vi "运维调试_氨氮.vi"() -> ()   [LabVIEW 2016, in "斯坦道氨氮.lvlib"]
uses:
  <vilib>/Utility/miscctls.llb/LVPointTypeDef.ctl
  <vilib>/Utility/config.llb/NI_LVConfig.lvlib
  <vilib>/ptbypt/NI_PtbyPt.lvlib
panel:
  in  "模块启用":bool
  in  "串口设置":bool
  in  "备用系数一键写入":bool
  in  "公式一键写入":bool
  in  "流程文件路径":path=path "C:/Users/Hsiao/Documents/斯坦道流程文件/流程.xml"
  in  "曲线模型":cluster{"X^2":dbl, "X":dbl, "B":dbl}(xcontrol)
  in  "质控参数设置":bool
  out "字符串":string
  in  "氨氮自动测试量程配置":T1
  out "ADC":sgl
  out "温度2":sgl
  out "温度1":sgl
  out "固件版本号":string
  in  "数组":string[](array[string])
  in  "备用系数写入":bool
  in  "备用系数读取":bool
  in  "备用系数":T2
  in  "量程切换阈值写入":bool
  in  "量程切换阈值读取":bool
  in  "量程切换阈值":cluster{"阈值":dbl, "标液浓度":dbl}
  in  "参数下拉列表":enum16{"氨氮", "总磷"}(ring)
  in  "量程下拉列表":enum16{"低量程", "高量程"}(ring)
  in  "测量模式下拉列表":enum16{"水样测量", "空白核查", "跨度核查", "标样核查", "加标回收"}(ring)
  in  "公式":cluster{"X^2":dbl, "X":dbl, "b":dbl}
  in  "写公式":bool
  in  "读公式":bool
  in  "返回":bool
  in  "设置":bool
  out "序列号":string="序列号"
  out "氨氮测量数据":T3(xcontrol)
  out "集成报警信息":string
  out "定时启动":bool
  out "总磷总氮运行状态":T4(xcontrol)
  in  "停止":bool
  in  "手动启动":bool
  in  "单步测试":bool
  in  "总磷氨氮调试":u16[](xcontrol)
  out "F3":sgl format="%#.6f"
  out "F2":sgl format="%#.6f"
  out "F1":sgl format="%#.6f"
  out "F0":sgl format="%#.6f"
  out "多列列表框":i32(listbox)
  # "参数设置"
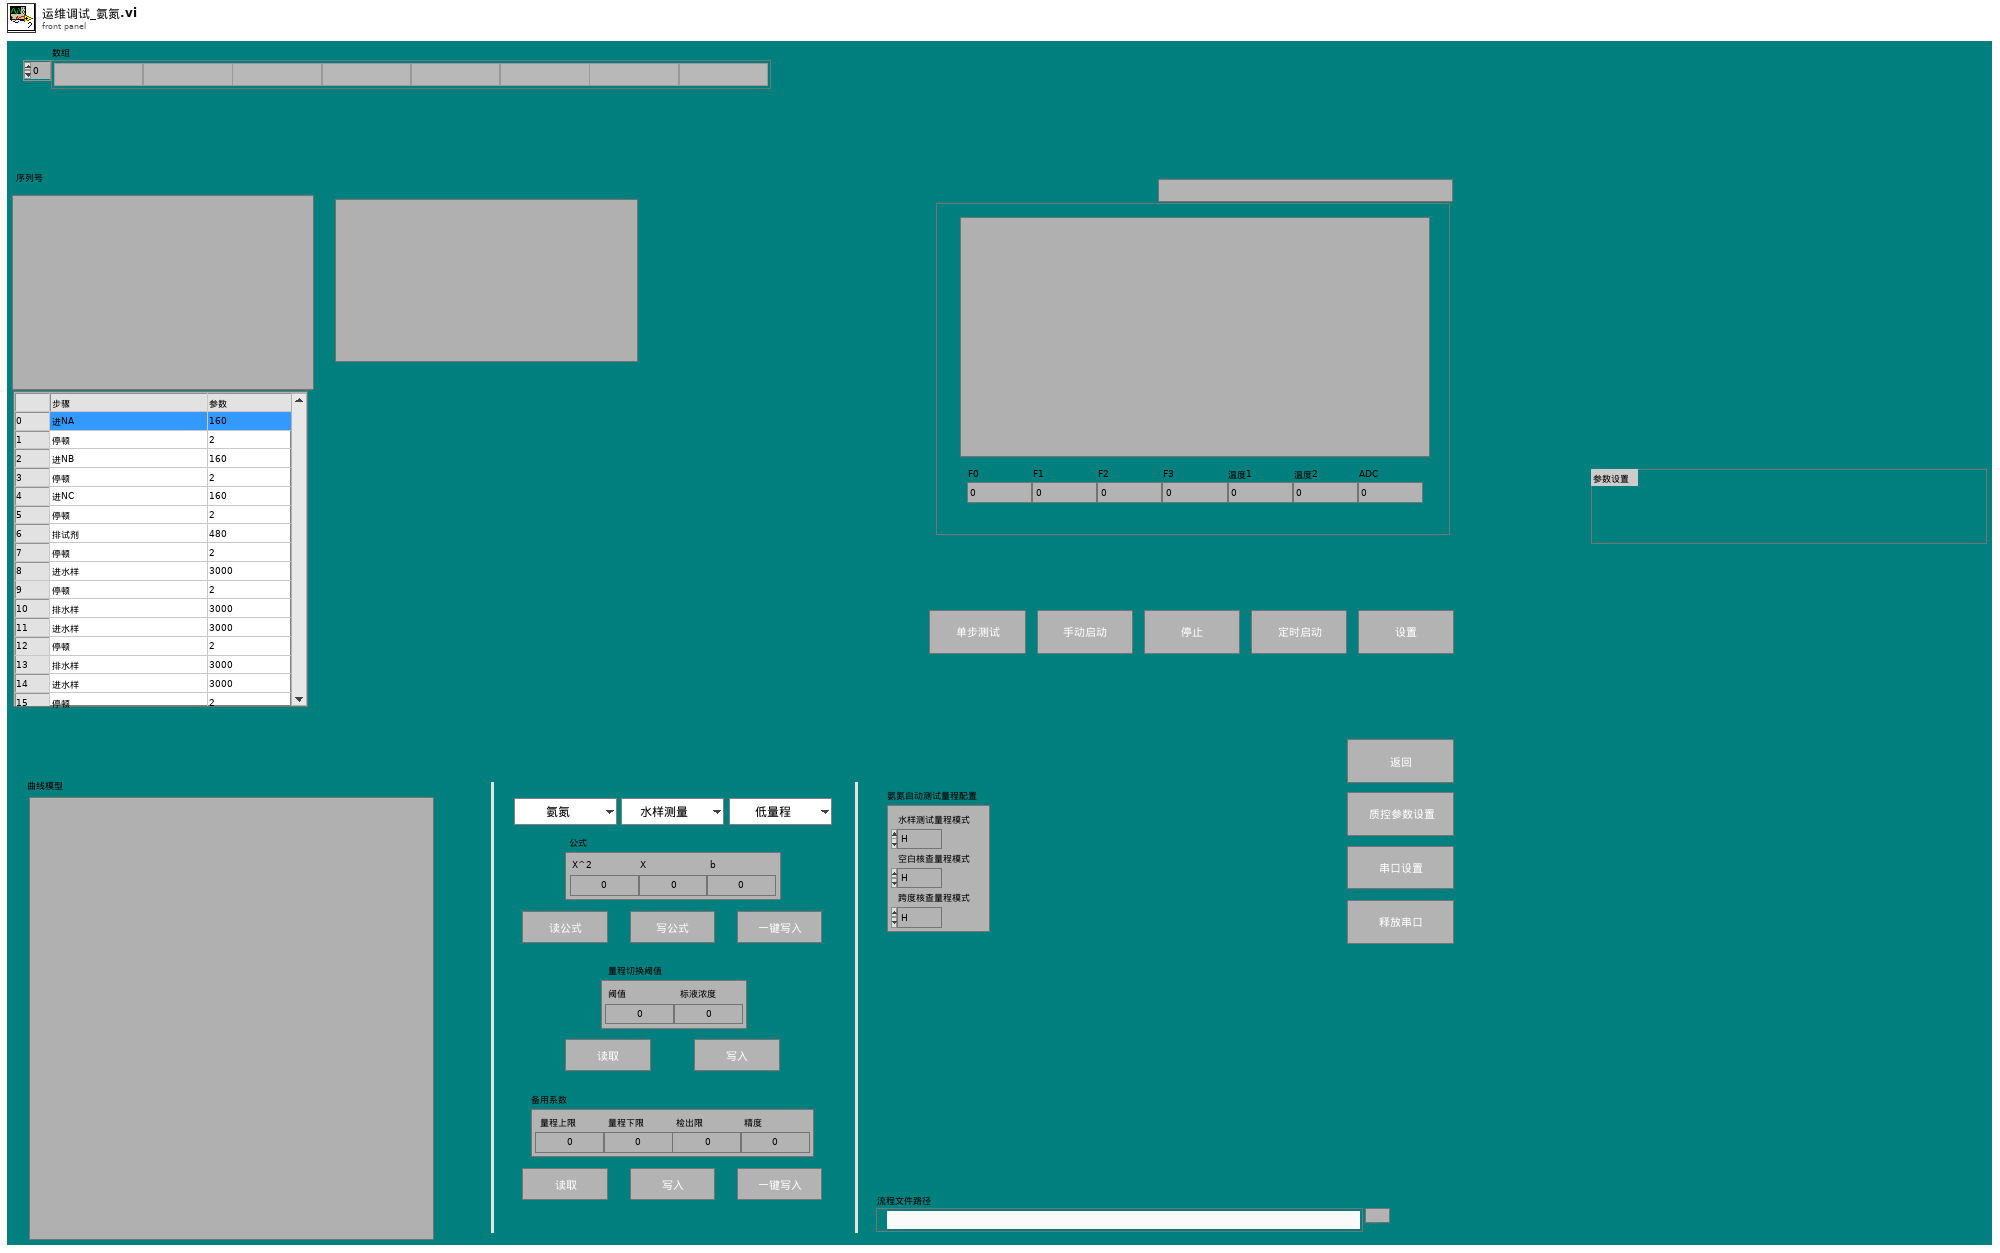
[diagram p1: front panel]
types:
  T1 = cluster{"水样测试量程模式":enum16{"H", "L", "AUTO"}, "空白核查量程模式":enum16{"H", "L", "AUTO"}, "跨度核查量程模式":enum16{"H", "L", "AUTO"}}
  T2 = cluster{"量程上限":dbl, "量程下限":dbl, "检出限":dbl, "精度":dbl}
  T3 = cluster{"flowid":u16, "测量精度":u16, "测量数据区":cluster{"因子编码":u32, "单位":u16, "标样参考值":sgl, "水样数据时间":timestamp, "水样实测值":sgl, "水样数据标识":string, "标样数据时间":timestamp, "标样实测值":sgl, "标样数据标识":string, "空白数据时间":timestamp, "空白实测值":sgl, "空白数据标识":string, "零点核查数据时间":timestamp, "零点核查实测值":sgl, "零点核查数据标识":string, "跨度核查数据时间":timestamp, "跨度核查实测值":sgl, "跨度核查数据标识":string, "加标回收数据时间":timestamp, "加标回收实测值":sgl, "加标回收数据标识":string, "平行样数据时间":timestamp, "平行样实测值":sgl, "平行样数据标识":string}}
  T4 = cluster{"系统时间":timestamp, "工作状态":enum16{"空闲", "水样测试", "标样核查", "零点核查", "跨度核查", "空白测试", "平行样测试", "加标回收", "空白校准", "标样校准", "初始化（清洗）"}, "测量模式":enum16{"待机", "连续模式", "周期模式", "定点模式", "受控模式", "手动模式"}, "告警代码":enum16{"无告警", "缺试剂告警", "缺水样告警", "缺蒸馏水告警", "缺标液告警", "仪表漏液告警", "标定异常告警", "超量程告警", "加热异常", "低试剂预警", "超上限告警", "超下限告警", "仪表内部其他异常", "滴定异常告警", "电极异常告警", "量程切换告警", "参数设置告警", "PH电极电位异常", "电导率电极异常", "浊度光度异常", "溶解氧电极异常", "溶解氧光强异常", "温度异常告警", "PH异常告警", "溶解氧异常告警", "电导率异常告警", "浊度异常告警", "叶绿素异常告警", "藻密度异常告警", "蓝绿藻异常告警", "ORP异常告警", "氨氮异常告警", "清洁刷异常告警", "SD卡异常告警", "蓝牙异常告警", "Wifi异常告警", "流程异常告警"}, "故障代码":enum16{"无故障", "电机故障", "温度故障", "通讯故障", "滴定故障"}, "日志代码":u16, "软件版本":u16, "F0":sgl, "F1":sgl, "F2":sgl, "F3":sgl, "T":sgl, "H":sgl, "id":u16, "flowid":u16, "量程":u16, "总磷控温温度1":sgl, "营养盐控温温度2":sgl, "ADC":sgl}
  T5 = cluster{"站号":u16, "量程切换":enum32{"H", "L", "AUTO"}, "控制命令":enum16{"启动测量", "标样核查", "零点核查", "跨度核查", "空白测试", "平行样测试", "加标回收", "空白校准", "标样校准", "初始化（清洗）", "停止测试", "仪器重启", "校时", "模式设置", "测量间隔设置"}, "模式设置":enum16{"待机", "连续模式", "周期模式", "定点模式", "受控模式", "手动模式"}, "测量间隔":u16}
  T6 = enum16{"启动测量", "标样核查", "零点核查", "跨度核查", "空白测试", "平行样测试", "加标回收", "空白校准", "标样校准", "初始化（清洗）", "停止测试", "仪器重启", "校时", "模式设置", "测量间隔设置"}
  T7 = cluster{"仪器测试类型":enum16{"水样测试", "标样核查", "空白测试", "跨度核查"}, "周期设置类型":enum16{"定点启动", "间隔启动"}, "定时功能启用":bool, "定时间隔":dbl, "24H周期设置":bool[]}
  T8 = enum32{"Bad", "Idle", "Run top level", "Running"}
  T9 = typedef "LVDateTimeRec.ctl" = cluster{"秒数的小数部分":dbl, "秒":i32, "分":i32, "时":i32, "日":i32, "月":i32, "年":i32, "天数（周）":i32, "天数（年）":i32, "DST":i32}
  T10 = typedef "LVPointTypeDef.ctl" = cluster{"Horizontal":i16, "Vertical":i16}
  T11 = cluster{"因子编码":u32, "单位":u16, "标样参考值":sgl, "水样数据时间":timestamp, "水样实测值":sgl, "水样数据标识":string, "标样数据时间":timestamp, "标样实测值":sgl, "标样数据标识":string, "空白数据时间":timestamp, "空白实测值":sgl, "空白数据标识":string, "零点核查数据时间":timestamp, "零点核查实测值":sgl, "零点核查数据标识":string, "跨度核查数据时间":timestamp, "跨度核查实测值":sgl, "跨度核查数据标识":string, "加标回收数据时间":timestamp, "加标回收实测值":sgl, "加标回收数据标识":string, "平行样数据时间":timestamp, "平行样实测值":sgl, "平行样数据标识":string}
  T12 = enum16{"空闲", "水样测试", "标样核查", "零点核查", "跨度核查", "空白测试", "平行样测试", "加标回收", "空白校准", "标样校准", "初始化（清洗）"}
  T13 = typedef "NI_LVConfig.lvlib/Config Data RefNum.ctl" = refnum<k1>
  T14 = cluster{"启动模式":enum16{"跨度核查", "水样测量", "空白核查", "标样核查", "加标回收"}, "启动参数":u16, "量程":enum16{"低量程", "高量程"}}
  T15 = cluster{"时间标识":timestamp, "设备":string, "日志信息":string, "流程参数":string}
  T16 = cluster{"时间标识":timestamp, "设备":string, "日志信息":string}
  T17 = enum16{"无告警", "缺试剂告警", "缺水样告警", "缺蒸馏水告警", "缺标液告警", "仪表漏液告警", "标定异常告警", "超量程告警", "加热异常", "低试剂预警", "超上限告警", "超下限告警", "仪表内部其他异常", "滴定异常告警", "电极异常告警", "量程切换告警", "参数设置告警", "PH电极电位异常", "电导率电极异常", "浊度光度异常", "溶解氧电极异常", "溶解氧光强异常", "温度异常告警", "PH异常告警", "溶解氧异常告警", "电导率异常告警", "浊度异常告警", "叶绿素异常告警", "藻密度异常告警", "蓝绿藻异常告警", "ORP异常告警", "氨氮异常告警", "清洁刷异常告警", "SD卡异常告警", "蓝牙异常告警", "Wifi异常告警", "流程异常告警"}
  T18 = typedef "LVRowAndColumnUnsignedTypeDef.ctl" = cluster{"Row":u32, "Column":u32}
  T19 = cluster{"跨度值":dbl, "零点标准液浓度":dbl, "跨度标准液浓度":dbl, "标准液标准浓度":dbl}
  T20 = cluster{"确定":bool, "跨度值":dbl, "零点标准液浓度":dbl, "跨度标准液浓度":dbl, "标准液标准浓度":dbl}
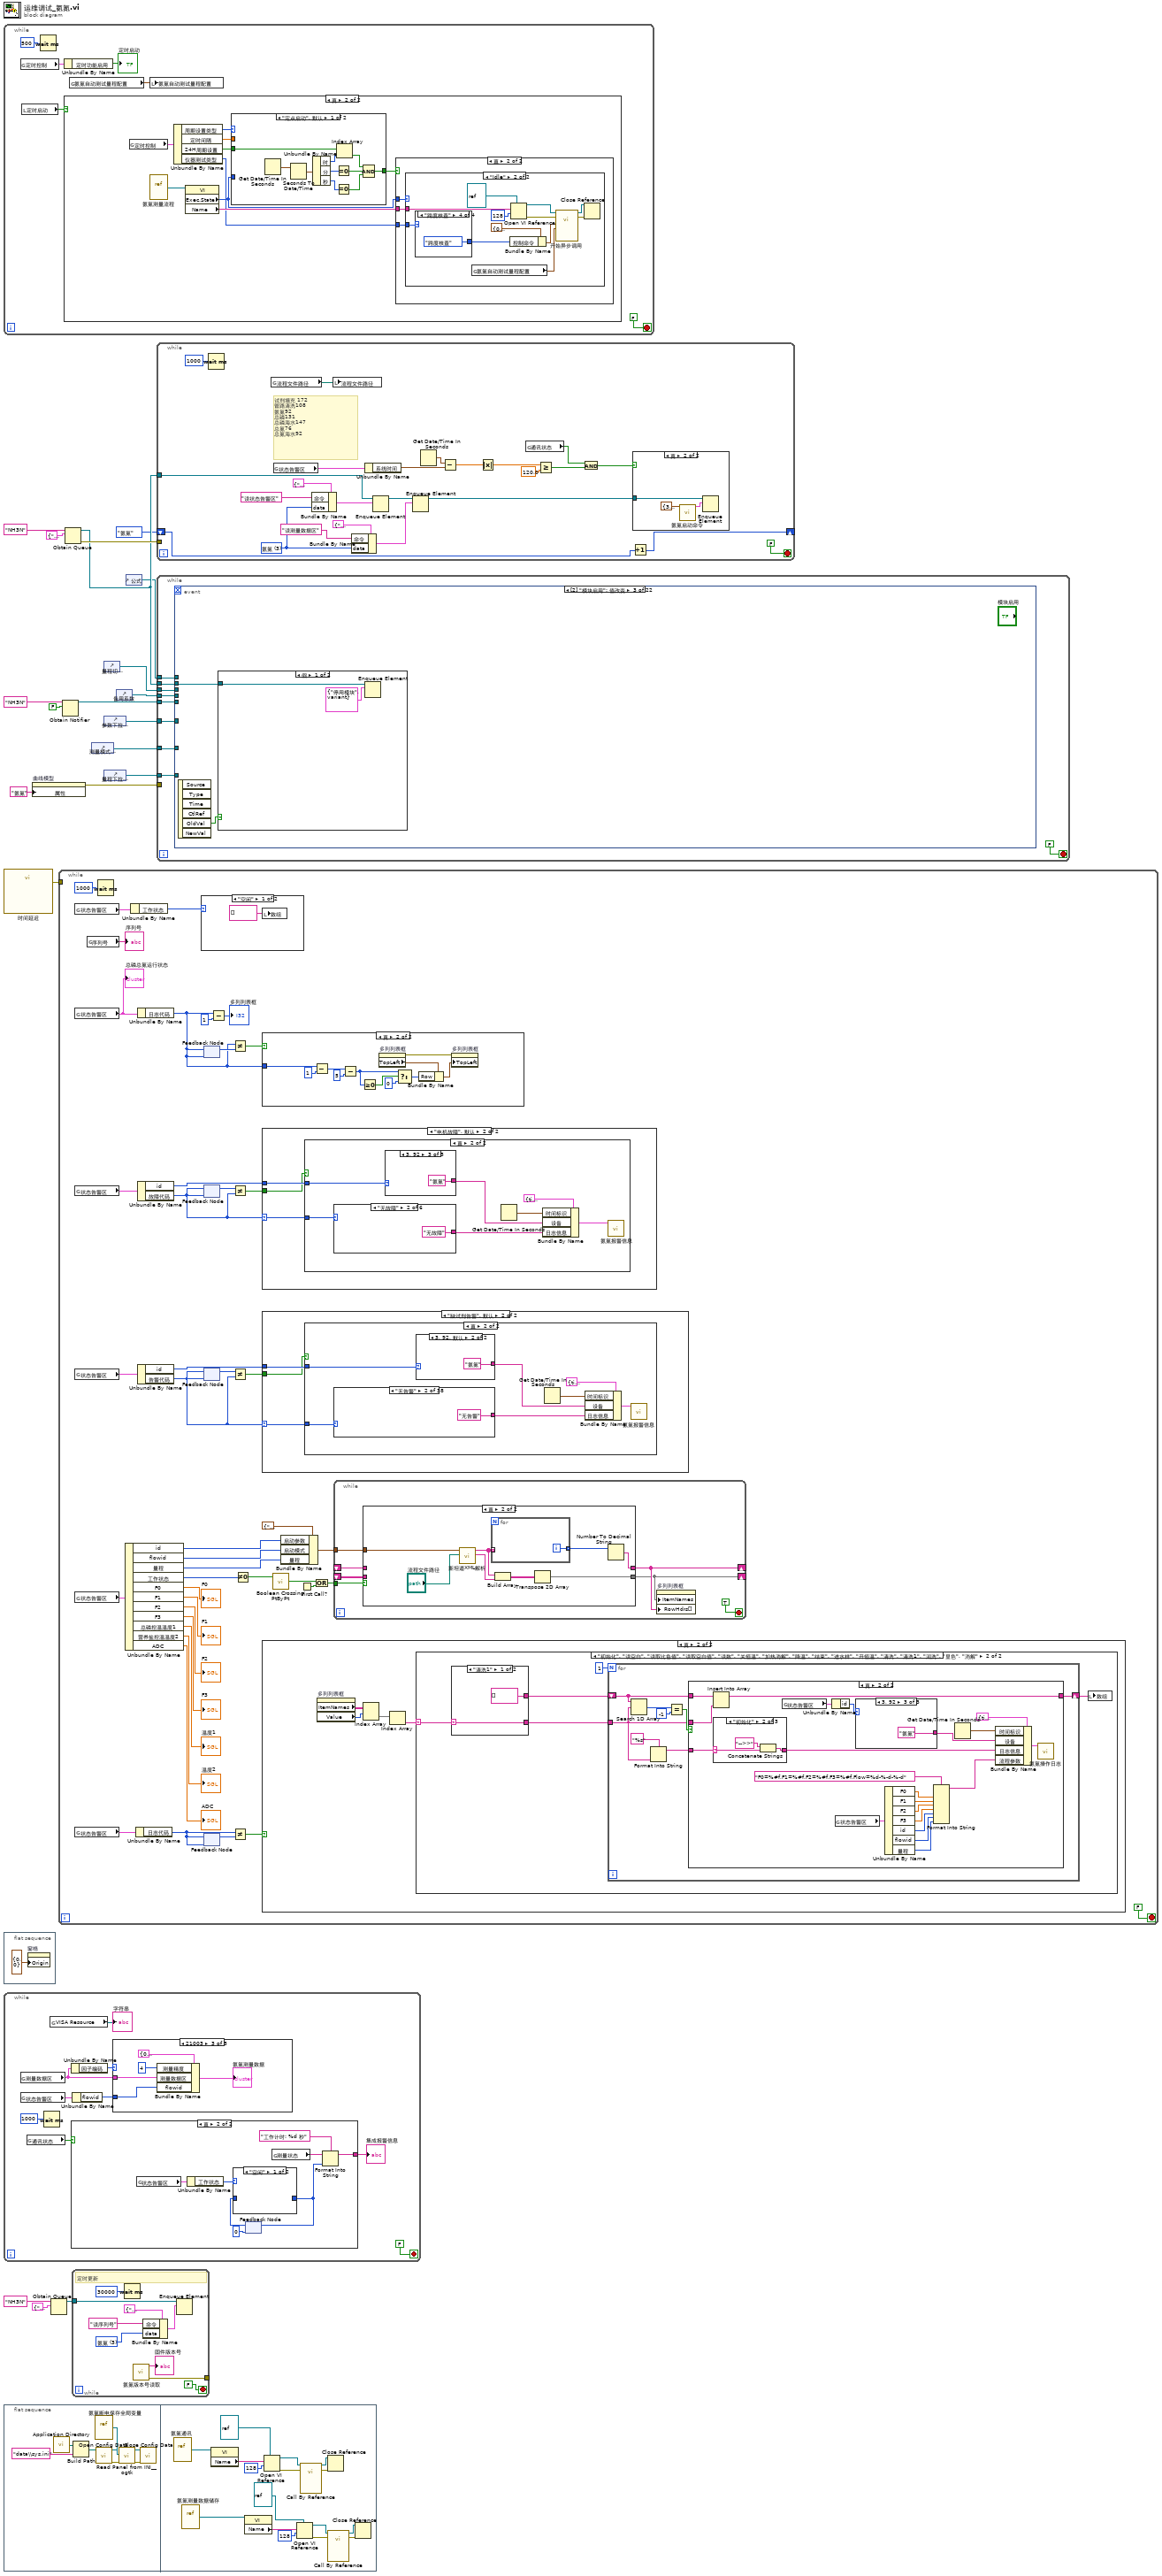
[diagram p0: block diagram]
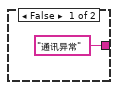
[diagram p2: hidden frame]
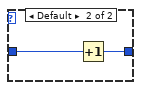
[diagram p3: hidden frame]
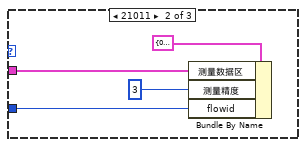
[diagram p5: hidden frame]
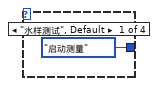
[diagram p9: hidden frame]
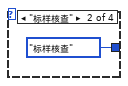
[diagram p10: hidden frame]
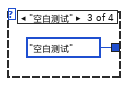
[diagram p11: hidden frame]
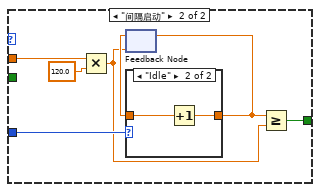
[diagram p12: hidden frame]
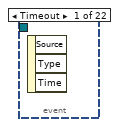
[diagram p14: hidden frame]
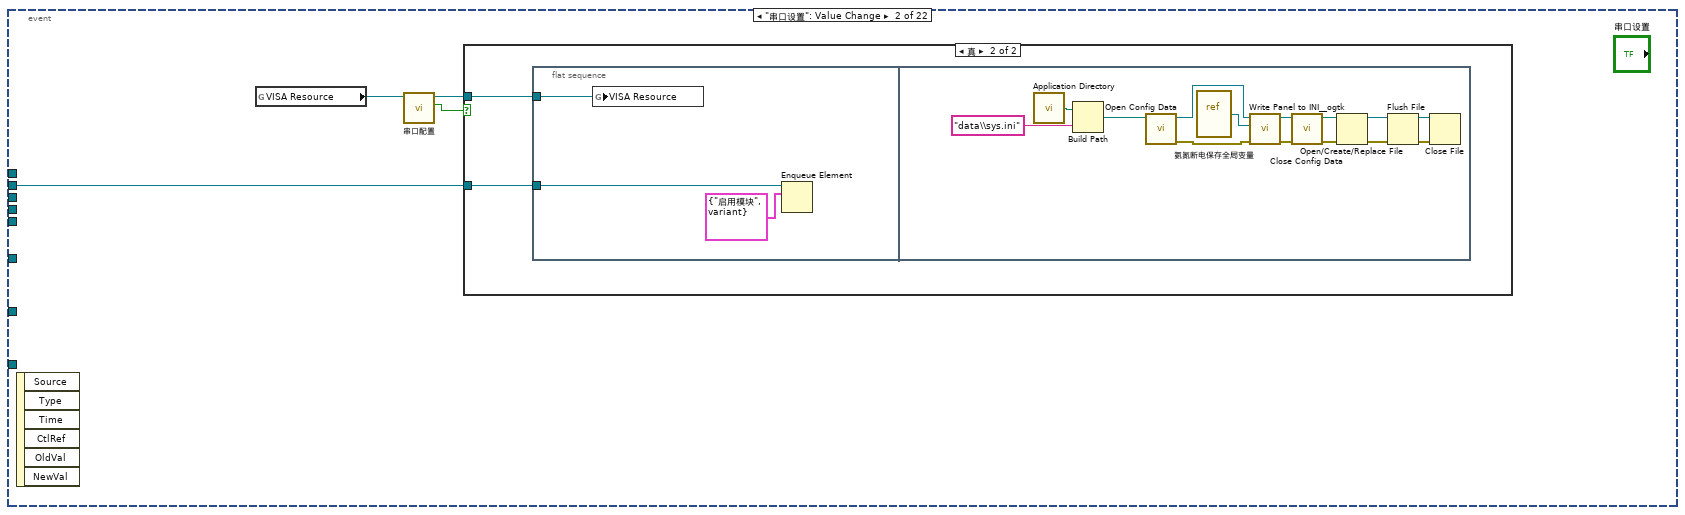
[diagram p15: hidden frame]
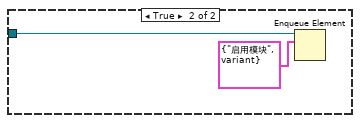
[diagram p17: hidden frame]
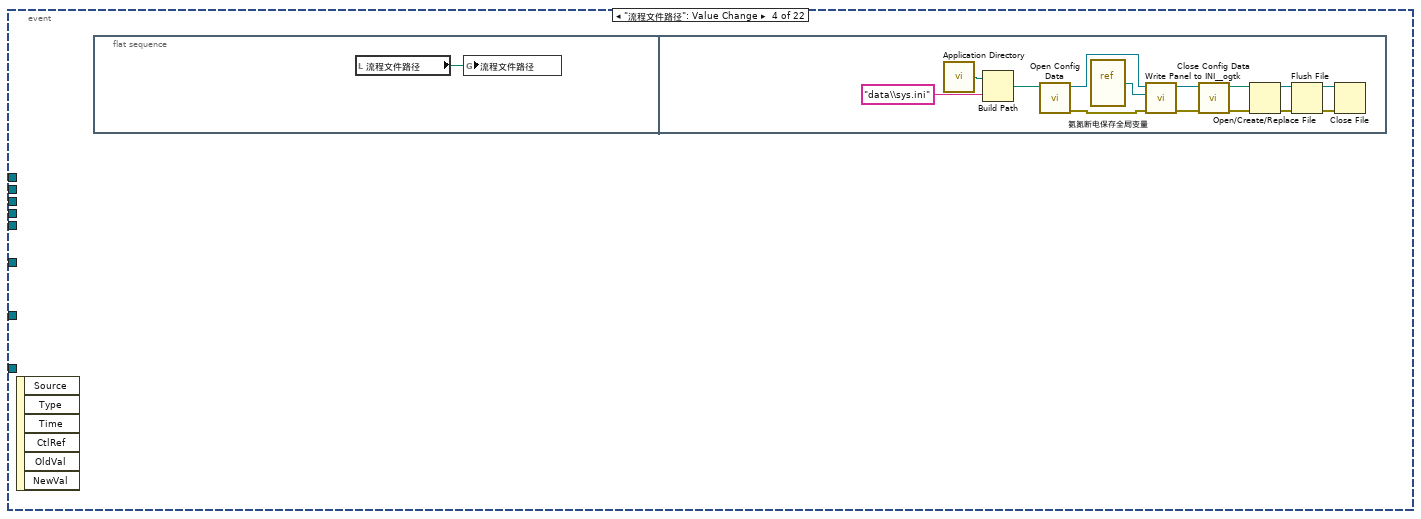
[diagram p18: hidden frame]
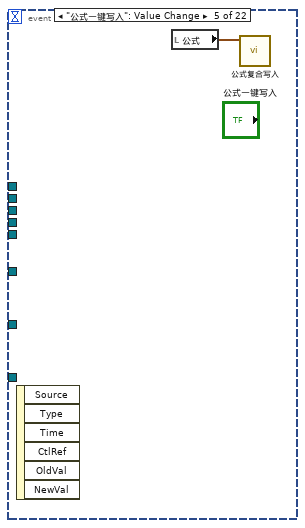
[diagram p19: hidden frame]
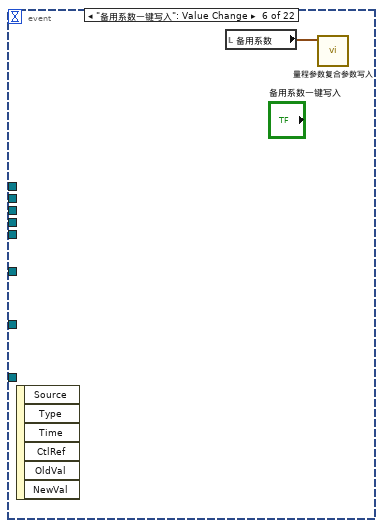
[diagram p20: hidden frame]
diagram:
  n1 = while {
    stop <- FALSE stop-if-true
    n2 = global read "氨氮断电保存全局变量.vi" "定时控制"() -> (w23:T7)
    n3 = local read "定时启动"() -> (w24:bool)
    n4 = Wait (ms)(milliseconds to wait=u32 500 ("等待时间（毫秒）")) -> ()  [unwired: 1 out]
    n5 = Unbundle By Name(w23) -> ("定时功能启用"=→"定时启动":bool)
    n6 = case shown="真" w24 {
      frame False {
      }
      frame True {
        n7 = global read "氨氮断电保存全局变量.vi" "定时控制"() -> (w35:T7)
        n8 = vi-ref "氨氮测量流程.vi"() -> (w31:refnum<vi>)
        n9 = Unbundle By Name(w35) -> ("周期设置类型"=w34:enum16{"定点启动", "间隔启动"}, "定时间隔"=w33:dbl, "24H周期设置"=w32:bool[], "仪器测试类型"=w28:enum16{"水样测试", "标样核查", "空白测试", "跨度核查"})
        n10 = property class="VI"(reference=w31) -> ("Exec.State"=w27:T8, "Name"=w30:string)  [unwired: 1 in, 2 out]
        n11 = case shown="\"定点启动\", 默认" w34 {
          tunnel: w33 -> [_ w68]
          tunnel: w32 -> [w64 _]
          tunnel: w27 -> [_ w71]
          tunnel: [w63 w66] -> w29
          frame "定点启动", Default {
            n12 = Get Date/Time In Seconds() -> (seconds since 1Jan1904=w62:timestamp)
            n13 = Seconds To Date/Time(time stamp (now)=w62) -> (date time rec=w61:T9)  [unwired: 1 in]
            n14 = Unbundle By Name(w61) -> ("时"=w60:i32, "分"=w58:i32, "秒"=w59:i32)
            n15 = Equal To 0?(x=w58) -> (x = 0?=w56:bool)
            n16 = Equal To 0?(x=w59) -> (x = 0?=w55:bool)
            n17 = Index Array(array=w64, index=w60) -> (element=w57:bool)
            n18 = Compound Arithmetic op=AND ("复合运算")(w57, w56, w55) -> (w63:bool)
          }
          frame "间隔启动" {
            n19 = Multiply(x=w68, y=120.0) -> (x*y=w65:dbl)
            n20 = feedback #1(w65) -> (w70:dbl)
            n21 = case shown="\"Idle\"" w71 {
              tunnel: w70 -> [_ w73]
              tunnel: [_ w72] -> w69
              frame "Bad", Default {
              }
              frame "Idle" {
                n22 = Increment(x=w73) -> (x+1=w72:dbl)
              }
            }
            n23 = feedback-in #1(w69) -> ()
            n24 = Greater Or Equal?(x=w69, y=w65) -> (x >= y?=w66:bool)
          }
        }
        n25 = case shown="真" w29 {
          tunnel: w30 -> [_ w38]
          tunnel: w28 -> [_ w37]
          tunnel: w27 -> [_ w36]
          frame False {
          }
          frame True {
            n26 = case shown="\"Idle\"" w36 {
              tunnel: w38 -> [_ w45]
              tunnel: w37 -> [_ w41]
              frame "Bad", Default {
              }
              frame "Idle" {
                n27 = case shown="\"跨度核查\"" w41 {
                  tunnel: [T6."启动测量" ("控制命令") T6."标样核查" ("控制命令") T6."空白测试" ("控制命令") T6."跨度核查" ("控制命令")] -> w40
                  frame "水样测试", Default {
                  }
                  frame "标样核查" {
                  }
                  frame "空白测试" {
                  }
                  frame "跨度核查" {
                  }
                }
                n28 = global read "氨氮断电保存全局变量.vi" "氨氮自动测试量程配置"() -> (w39:T1)
                n29 = Bundle By Name(cluster=T5 {"站号"=0, "量程切换"=enum."H", "控制命令"=enum."启动测量", "模式设置"=enum."待机", "测量间隔"=0} ("参数"), "控制命令"=w40) -> (w42:T5)
                n30 = Open VI Reference(type specifier VI Refnum (for type only)=refnum<vi> refnum, vi path=w45, options=128 ("选项")) -> (vi reference=w46:refnum<vi>, error out=w47:errorcluster)  [unwired: 3 in]
                n31 = call-by-ref "开始异步调用"(reference=w46, error in=w47, "量程模式"=w39, "参数"=w42) -> (reference out=w48:refnum<vi>, error out=w49:errorcluster)  [unwired: 10 in]
                n32 = Close Reference(reference=w48, error in (no error)=w49) -> ()  [unwired: 1 out]
              }
            }
          }
        }
      }
    }
    n33 = global read "氨氮断电保存全局变量.vi" "氨氮自动测试量程配置"() -> (w21:T1)
    n34 = local write "氨氮自动测试量程配置"(w21) -> ()
  }
  n35 = call "时间延迟"() -> ("error out"=w9:errorcluster)  [unwired: 11 in]
  n36 = flat-sequence {
    frame #0 {
      n37 = property on="窗格" class="Pane"("Origin"=T10 {"Horizontal"=0, "Vertical"=0} ("原点")) -> ()  [unwired: 2 in, 2 out]
    }
  }
  n38 = while {
    stop <- FALSE stop-if-true
    n39 = global read "VAR氨氮全局变量.vi" "测量数据区"() -> (w81:T11)
    n40 = global read "VAR氨氮全局变量.vi" "状态告警区"() -> (w77:T4)
    n41 = global read "VAR氨氮全局变量.vi" "通讯状态"() -> (w79:bool)
    n42 = Wait (ms)(milliseconds to wait=u32 1000 ("等待时间（毫秒）")) -> ()  [unwired: 1 out]
    n43 = global read "氨氮断电保存全局变量.vi" "VISA Resource"() -> (→"字符串":refnum<visa-resource-name>)
    n44 = Unbundle By Name(w81) -> ("因子编码"=w80:u32)
    n45 = case shown="真" w79 {
      tunnel: ["通讯异常" ("集成报警信息") w86] -> w78
      frame False {
      }
      frame True {
        n46 = global read "VAR氨氮全局变量.vi" "状态告警区"() -> (w92:T4)
        n47 = Unbundle By Name(w92) -> ("工作状态"=w91:T12)
        n48 = feedback #2(0) -> (w89:i32)
        n49 = case shown="\"空闲\"" w91 {
          tunnel: w89 -> [_ w94]
          tunnel: [_ w93] -> w87
          frame "空闲" {
          }
          frame Default {
            n50 = Increment(x=w94) -> (x+1=w93:i32)
          }
        }
        n51 = feedback-in #2(w87) -> ()
        n52 = global read "VAR氨氮全局变量.vi" "测量状态"() -> (w85:string)
        n53 = Format Into String(format string="工作计时: %d 秒" ("格式字符串"), initial string=w85, w87) -> (resulting string=w86:string)  [unwired: 1 in, 1 out]
      }
    }
    "集成报警信息" <- w78
    n54 = Unbundle By Name(w77) -> ("flowid"=w76:u16)
    n55 = case shown="21003" w80 {
      tunnel: w81 -> [_ w98 w103]
      tunnel: w76 -> [_ w96 w101]
      frame Default {
      }
      frame 21011 {
        n56 = Bundle By Name(cluster=T3 {"flowid"=0, "测量精度"=0, "测量数据区"={"因子编码"=0, "单位"=0, "标样参考值"=0.0, "水样数据时间"=timestamp(0 s since 1904-01-01), "水样实测值"=0.0, "水样数据标识"="", "标样数据时间"=timestamp(0 s since 1904-01-01), "标样实测值"=0.0, "标样数据标识"="", "空白数据时间"=timestamp(0 s since 1904-01-01), "空白实测值"=0.0, "空白数据标识"="", "零点核查数据时间"=timestamp(0 s since 1904-01-01), "零点核查实测值"=0.0, "零点核查数据标识"="", "跨度核查数据时间"=timestamp(0 s since 1904-01-01), "跨度核查实测值"=0.0, "跨度核查数据标识"="", "加标回收数据时间"=timestamp(0 s since 1904-01-01), "加标回收实测值"=0.0, "加标回收数据标识"="", "平行样数据时间"=timestamp(0 s since 1904-01-01), "平行样实测值"=0.0, "平行样数据标识"=""}} ("氨氮测量数据"), "测量数据区"=w98, "测量精度"=u16 3, "flowid"=w96) -> ()  [unwired: 1 out]
      }
      frame 21003 {
        n57 = Bundle By Name(cluster=T3 {"flowid"=0, "测量精度"=0, "测量数据区"={"因子编码"=0, "单位"=0, "标样参考值"=0.0, "水样数据时间"=timestamp(0 s since 1904-01-01), "水样实测值"=0.0, "水样数据标识"="", "标样数据时间"=timestamp(0 s since 1904-01-01), "标样实测值"=0.0, "标样数据标识"="", "空白数据时间"=timestamp(0 s since 1904-01-01), "空白实测值"=0.0, "空白数据标识"="", "零点核查数据时间"=timestamp(0 s since 1904-01-01), "零点核查实测值"=0.0, "零点核查数据标识"="", "跨度核查数据时间"=timestamp(0 s since 1904-01-01), "跨度核查实测值"=0.0, "跨度核查数据标识"="", "加标回收数据时间"=timestamp(0 s since 1904-01-01), "加标回收实测值"=0.0, "加标回收数据标识"="", "平行样数据时间"=timestamp(0 s since 1904-01-01), "平行样实测值"=0.0, "平行样数据标识"=""}} ("氨氮测量数据"), "测量精度"=u16 4, "测量数据区"=w103, "flowid"=w101) -> (→"氨氮测量数据":T3)
      }
    }
  }
  n58 = flat-sequence {
    frame #0 {
      n59 = call <vilib>:"Application Directory.vi"() -> ("Application Directory"=w104:path)
      n60 = Build Path(base path=w104, name or relative path="data\\sys.ini" ("名称或相对路径")) -> (appended path=w106:path)
      n61 = vi-ref "氨氮断电保存全局变量.vi"() -> (w108:refnum<vi>)
      n62 = call <vilib>:"Open Config Data.vi"("configuration file path"=w106) -> ("error out"=w110:errorcluster, "refnum"=w107:T13)  [unwired: 8 in, 1 out]
      n63 = call <userlib>:"Read Panel from INI__ogtk.vi"("error in (no error)"=w110, "VI ref"=w108, "refnum"=w107) -> ("error out"=w111:errorcluster, "refnum out"=w109:T13)  [unwired: 7 in]
      n64 = call <vilib>:"Close Config Data.vi"("error in (no error)"=w111, "refnum"=w109) -> ()  [unwired: 8 in, 2 out]
    }
    frame #1 {
      n65 = vi-ref "氨氮通讯.vi"() -> (w127:refnum<vi>)
      n66 = vi-ref "氨氮测量数据储存.vi"() -> (w119:refnum<vi>)
      n67 = property class="VI"(reference=w127) -> ("Name"=w126:string)  [unwired: 1 in, 2 out]
      n68 = property class="VI"(reference=w119) -> ("Name"=w112:string)  [unwired: 1 in, 2 out]
      n69 = Open VI Reference(type specifier VI Refnum (for type only)=refnum<vi> refnum, vi path=w126, options=128 ("选项")) -> (vi reference=w124:refnum<vi>, error out=w122:errorcluster)  [unwired: 3 in]
      n70 = Open VI Reference(type specifier VI Refnum (for type only)=refnum<vi> refnum, vi path=w112, options=128 ("选项")) -> (vi reference=w114:refnum<vi>, error out=w116:errorcluster)  [unwired: 3 in]
      n71 = call-by-ref "?"(reference=w124, error in=w122) -> (reference out=w120:refnum<vi>, error out=w121:errorcluster)  [unwired: 12 in]
      n72 = Close Reference(reference=w120, error in (no error)=w121) -> ()  [unwired: 1 out]
      n73 = call-by-ref "?"(reference=w114, error in=w116) -> (reference out=w118:refnum<vi>, error out=w117:errorcluster)  [unwired: 12 in]
      n74 = Close Reference(reference=w118, error in (no error)=w117) -> ()  [unwired: 1 out]
    }
  }
  n75 = property on="曲线模型" class="氨氮曲线模型 (严格)"("属性"="氨氮" ("调用模块名称属性")) -> (error out=w2:errorcluster)  [unwired: 2 in, 1 out]
  n76 = Obtain Queue(name (unnamed)="NH3N" ("名称（未命名）"), element data type=cluster{"命令":string, "data":variant} {"命令"="", "data"=variant}) -> (queue out=w6:refnum<queue>)  [unwired: 3 in, 2 out]
  n77 = while {
    tunnel: w9 -> [_]
    stop <- FALSE stop-if-true
    n78 = global read "VAR氨氮全局变量.vi" "状态告警区"() -> (w143:T4)
    n79 = global read "VAR氨氮全局变量.vi" "状态告警区"() -> (w155:T4)
    "总磷总氮运行状态" <- w155
    n80 = global read "VAR氨氮全局变量.vi" "状态告警区"() -> (w148:T4)
    n81 = global read "VAR氨氮全局变量.vi" "状态告警区"() -> (w153:T4)
    n82 = global read "VAR氨氮全局变量.vi" "状态告警区"() -> (w163:T4)
    n83 = global read "VAR氨氮全局变量.vi" "状态告警区"() -> (w140:T4)
    n84 = global read "VAR氨氮全局变量.vi" "序列号"() -> (→"序列号":string)
    n85 = Wait (ms)(milliseconds to wait=u32 1000 ("等待时间（毫秒）")) -> ()  [unwired: 1 out]
    n86 = Unbundle By Name(w163) -> ("id"=w160:u16, "flowid"=w162:u16, "量程"=w161:u16, "工作状态"=w129:T12, "F0"=→"F0":sgl, "F1"=→"F1":sgl, "F2"=→"F2":sgl, "F3"=→"F3":sgl, "总磷控温温度1"=→"温度1":sgl, "营养盐控温温度2"=→"温度2":sgl, "ADC"=→"ADC":sgl)
    n87 = Unbundle By Name(w143) -> ("工作状态"=w142:T12)
    n88 = Unbundle By Name(w140) -> ("日志代码"=w139:u16)
    n89 = Unbundle By Name(w155) -> ("日志代码"=w133:u16)
    n90 = Unbundle By Name(w148) -> ("id"=w147:u16, "故障代码"=w144:enum16{"无故障", "电机故障", "温度故障", "通讯故障", "滴定故障"})
    n91 = Unbundle By Name(w153) -> ("id"=w152:u16, "告警代码"=w149:T17)
    n92 = case shown="\"空闲\"" w142 {
      frame "空闲" {
        n93 = local write "数组"(string[] [] ("数组")) -> ()
      }
      frame "水样测试", Default {
      }
    }
    n94 = feedback-in #3(w133) -> ()
    n95 = feedback #3(w133) -> (w168:u16)
    n96 = feedback #4(w144) -> (w145:enum16{"无故障", "电机故障", "温度故障", "通讯故障", "滴定故障"})
    n97 = feedback-in #4(w144) -> ()
    n98 = feedback #5(w149) -> (w150:T17)
    n99 = feedback-in #5(w149) -> ()
    n100 = feedback #6(w139) -> (w141:u16)
    n101 = feedback-in #6(w139) -> ()
    n102 = Subtract(x=w133, y=1) -> (x-y=→"多列列表框":i32)
    n103 = Not Equal?(x=w133, y=w168) -> (x != y?=w167:bool)
    n104 = Not Equal?(x=w145, y=w144) -> (x != y?=w146:bool)
    n105 = Not Equal?(x=w150, y=w149) -> (x != y?=w151:bool)
    n106 = Not Equal?(x=w139, y=w141) -> (x != y?=w138:bool)
    n107 = Not Equal To 0?(x=w129) -> (x != 0?=w165:bool)
    n108 = case shown="真" w167 {
      tunnel: w133 -> [_ w318]
      frame False {
      }
      frame True {
        n109 = Subtract(x=w318, y=1) -> (x-y=w316:i32)
        n110 = Subtract(x=w316, y=5) -> (x-y=w320:i32)
        n111 = Greater Or Equal To 0?(x=w320) -> (x >= 0?=w319:bool)
        n112 = property on="多列列表框" class="MCListbox (严格)"() -> (error out=w324:errorcluster, "TopLeft"=w325:T18)  [unwired: 2 in, 1 out]
        n113 = Select(t=w320, s=w319, f=0) -> (s? t:f=w321:i32)
        n114 = Bundle By Name(cluster=w325, "Row"=w321) -> (w326:T18)
        n115 = property on="多列列表框" class="MCListbox (严格)"(error in=w324, "TopLeft"=w326) -> ()  [unwired: 1 in, 2 out]
      }
    }
    n116 = case shown="\"电机故障\", 默认" w144 {
      selector: w144 -> [_ w225]
      tunnel: w147 -> [_ w226]
      tunnel: w146 -> [_ w224]
      frame "无故障" {
      }
      frame "电机故障", Default {
        n117 = case shown="真" w224 {
          tunnel: w226 -> [_ w233]
          tunnel: w225 -> [_ w228]
          frame False {
          }
          frame True {
            n118 = case shown="\"无故障\"" w228 {
              selector: w228 -> [w235 _ _ _ _ _]
              tunnel: [w234 "无故障" "电机故障" "温度故障" "通讯故障" "滴定故障"] -> w227
              frame Default {
                n119 = Format Into String(format string="%d" ("格式字符串"), initial string="未知" ("工作状态"), w235) -> (resulting string=w234:string)  [unwired: 1 in, 1 out]
              }
              frame "无故障" {
              }
              frame "电机故障" {
              }
              frame "温度故障" {
              }
              frame "通讯故障" {
              }
              frame "滴定故障" {
              }
            }
            n120 = case shown="3, 92" w233 {
              tunnel: [_ "总磷" ("table输入") "氨氮" ("table输入")] -> w229
              frame Default {
              }
              frame 1, 131 {
              }
              frame 3, 92 {
              }
            }
            n121 = Get Date/Time In Seconds() -> (seconds since 1Jan1904=w230:timestamp)
            n122 = Bundle By Name(cluster=T16 {"时间标识"=timestamp(0 s since 1904-01-01), "设备"="", "日志信息"=""} ("data in"), "时间标识"=w230, "设备"=w229, "日志信息"=w227) -> (w231:T16)
            n123 = call "氨氮报警信息.vi"("data in"=w231) -> ()  [unwired: 11 in]
          }
        }
      }
    }
    n124 = case shown="\"缺试剂告警\", 默认" w149 {
      selector: w149 -> [_ w246]
      tunnel: w152 -> [_ w247]
      tunnel: w151 -> [_ w245]
      frame "无告警" {
      }
      frame "缺试剂告警", Default {
        n125 = case shown="真" w245 {
          tunnel: w247 -> [_ w254]
          tunnel: w246 -> [_ w248]
          frame False {
          }
          frame True {
            n126 = case shown="\"无告警\"" w248 {
              selector: w248 -> [w256 _ _ _ _ _ _ _ _ _ _ _ _ _ _ _ _ _ _ _ _ _ _ _ _ _ _ _ _ _ _ _ _ _ _ _ _ _]
              tunnel: [w255 "无告警" "缺试剂告警" "缺水样告警" "缺蒸馏水告警" "缺标液告警" "仪表漏液告警" "标定异常告警" "超量程告警" "加热异常" "低试剂预警" "超上限告警" "超下限告警" "仪表内部其他异常" "滴定异常告警" "电极异常告警" "量程切换告警" "参数设置告警" "PH电极电位异常" "电导率电极异常" "浊度光度异常" "溶解氧电极异常" "溶解氧光强异常" "温度异常告警" "PH异常告警" "溶解氧异常告警" "电导率异常告警" "浊度异常告警" "叶绿素异常告警" "藻密度异常告警" "蓝绿藻异常告警" "ORP异常告警" "氨氮异常告警" "清洁刷异常告警" "SD卡异常告警" "蓝牙异常告警" "WiFi异常告警" "流程异常告警"] -> w249
              frame Default {
                n127 = Format Into String(format string="%d" ("格式字符串"), initial string="未知" ("工作状态"), w256) -> (resulting string=w255:string)  [unwired: 1 in, 1 out]
              }
              frame "无告警" {
              }
              frame "缺试剂告警" {
              }
              frame "缺水样告警" {
              }
              frame "缺蒸馏水告警" {
              }
              frame "缺标液告警" {
              }
              frame "仪表漏液告警" {
              }
              frame "标定异常告警" {
              }
              frame "超量程告警" {
              }
              frame "加热异常" {
              }
              frame "低试剂预警" {
              }
              frame "超上限告警" {
              }
              frame "超下限告警" {
              }
              frame "仪表内部其他异常" {
              }
              frame "滴定异常告警" {
              }
              frame "电极异常告警" {
              }
              frame "量程切换告警" {
              }
              frame "参数设置告警" {
              }
              frame "PH电极电位异常" {
              }
              frame "电导率电极异常" {
              }
              frame "浊度光度异常" {
              }
              frame "溶解氧电极异常" {
              }
              frame "溶解氧光强异常" {
              }
              frame "温度异常告警" {
              }
              frame "PH异常告警" {
              }
              frame "溶解氧异常告警" {
              }
              frame "电导率异常告警" {
              }
              frame "浊度异常告警" {
              }
              frame "叶绿素异常告警" {
              }
              frame "藻密度异常告警" {
              }
              frame "蓝绿藻异常告警" {
              }
              frame "ORP异常告警" {
              }
              frame "氨氮异常告警" {
              }
              frame "清洁刷异常告警" {
              }
              frame "SD卡异常告警" {
              }
              frame "蓝牙异常告警" {
              }
              frame "Wifi异常告警" {
              }
              frame "流程异常告警" {
              }
            }
            n128 = case shown="3, 92, 默认" w254 {
              tunnel: ["总磷" ("table输入") "氨氮" ("table输入")] -> w250
              frame 1, 131 {
              }
              frame 3, 92, Default {
              }
            }
            n129 = Get Date/Time In Seconds() -> (seconds since 1Jan1904=w251:timestamp)
            n130 = Bundle By Name(cluster=T16 {"时间标识"=timestamp(0 s since 1904-01-01), "设备"="", "日志信息"=""} ("data in"), "时间标识"=w251, "设备"=w250, "日志信息"=w249) -> (w252:T16)
            n131 = call "氨氮报警信息.vi"("data in"=w252) -> ()  [unwired: 11 in]
          }
        }
      }
    }
    n132 = case shown="真" w138 {
      frame False {
      }
      frame True {
        n133 = property on="多列列表框" class="MCListbox (严格)"() -> ("ItemNames"=w174:string[][], "Value"=w175:i32)  [unwired: 2 in, 2 out]
        n134 = Index Array(array=w174, index (row)=w175) -> (element=w173:string[])  [unwired: 1 in]
        n135 = Index Array(array=w173) -> (element=w172:string)  [unwired: 1 in]
        n136 = case shown="\"初始化\", \"读空白\", \"读取比色值\", \"读取空白值\", \"读数\", \"关恒温\", \"加热消解\", \"降温\", \"结束\", \"进水样\", \"开恒温\", \"清洗\", \"清洗1\", \"润洗\", \"显色\", \"消解\"" w172 {
          selector: w172 -> [_ w178]
          frame Default {
          }
          frame "初始化", "读空白", "读取比色值", "读取空白值", "读数", "关恒温", "加热消解", "降温", "结束", "进水样", "开恒温", "清洗", "清洗1", "润洗", "显色", "消解" {
            n137 = case shown="\"清洗1\"" w178 {
              selector: w178 -> [w182 w184]
              tunnel: [w182 w184] -> w177
              tunnel: [string[] [] ("数组") "数组"] -> w176
              frame "清洗1" {
              }
              frame Default {
              }
            }
            n138 = for {
              N: 1 -> [_]
              tunnel: w177 -> [w186]
              shift-right: [w185] -> w179
              shift-left: w176 -> [w187]
              n139 = Search 1D Array(1D array=w187, element=w186) -> (index of element=w190:i32)  [unwired: 1 in]
              n140 = Format Into String(format string="%s" ("格式字符串"), w186) -> (resulting string=w191:string)  [unwired: 2 in, 1 out]
              n141 = Equal?(x=w190, y=-1) -> (x = y?=w188:bool)
              n142 = case shown="真" w188 {
                tunnel: w191 -> [_ w195]
                tunnel: w187 -> [w193 w199]
                tunnel: w186 -> [_ w198]
                tunnel: [w193 w197] -> w185
                frame False {
                }
                frame True {
                  n143 = Insert Into Array(array=w199, new element=w198) -> (w197:string[])  [unwired: 1 in]
                  n144 = case shown="\"初始化\"" w195 {
                    selector: w195 -> [w215 w218 w221]
                    tunnel: [w215 w217 w220] -> w194
                    frame Default {
                    }
                    frame "初始化" {
                      n145 = Concatenate Strings("-->>" ("字符串"), w218) -> (w217:string)
                    }
                    frame "结束" {
                      n146 = Concatenate Strings("-->>" ("字符串"), w221) -> (w220:string)
                    }
                  }
                  n147 = global read "VAR氨氮全局变量.vi" "状态告警区"() -> (w214:T4)
                  n148 = Unbundle By Name(w214) -> ("id"=w213:u16)
                  n149 = global read "VAR氨氮全局变量.vi" "状态告警区"() -> (w209:T4)
                  n150 = case shown="3, 92" w213 {
                    tunnel: [_ "总磷" ("table输入") "氨氮" ("table输入")] -> w211
                    frame Default {
                    }
                    frame 1, 131 {
                    }
                    frame 3, 92 {
                    }
                  }
                  n151 = Unbundle By Name(w209) -> ("F0"=w206:sgl, "F1"=w205:sgl, "F2"=w204:sgl, "F3"=w203:sgl, "id"=w202:u16, "flowid"=w201:u16, "量程"=w200:u16)
                  n152 = Format Into String(format string="F0=%#f,F1=%#f,F2=%#f,F3=%#f,Flow=%d-%-d-%-d" ("格式字符串"), w206, w205, w204, w203, w202, w201, w200) -> (resulting string=w207:string)  [unwired: 2 in, 1 out]
                  n153 = Get Date/Time In Seconds() -> (seconds since 1Jan1904=w210:timestamp)
                  n154 = Bundle By Name(cluster=T15 {"时间标识"=timestamp(0 s since 1904-01-01), "设备"="", "日志信息"="", "流程参数"=""} ("data in"), "时间标识"=w210, "设备"=w211, "日志信息"=w194, "流程参数"=w207) -> (w212:T15)
                  n155 = call "氨氮操作日志.vi"("data in"=w212) -> ()  [unwired: 11 in]
                }
              }
            }
            n156 = local write "数组"(w179) -> ()
          }
        }
      }
    }
    n157 = call <vilib>:"Boolean Crossing PtByPt.vi"("input"=w165) -> ("crossing"=w128:bool)  [unwired: 2 in]
    n158 = Bundle By Name(cluster=T14 {"启动模式"=enum."跨度核查", "启动参数"=1, "量程"=enum."低量程"} ("参数簇"), "启动参数"=w160, "启动模式"=w162, "量程"=w161) -> (w130:T14)
    n159 = First Call?() -> (First Call?: T/F=w166:bool)
    n160 = Or(x=w128, y=w166) -> (x .or. y?=w164:bool)
    n161 = while {
      tunnel: w164 -> [w304]
      tunnel: w130 -> [w303]
      shift-right: [w298] -> _
      shift-left: _ -> [w300]
      shift-right: [w299] -> _
      shift-left: _ -> [w301]
      stop <- TRUE stop-if-true
      n162 = case shown="真" w304 {
        tunnel: [w306 w314] -> w299
        tunnel: [w305 w313] -> w298
        tunnel: w303 -> [_ w308]
        tunnel: w301 -> [w306 _]
        tunnel: w300 -> [w305 _]
        frame False {
        }
        frame True {
          n163 = call "斯坦道XML解析.vi"("添加的路径"="流程文件路径", "参数簇"=w308) -> ("步骤时间"=w309:string[], "步骤名"=w311:string[])  [unwired: 8 in]
          n164 = for {
            tunnel: w311 -> [_] mode=indexing
            tunnel: [w315] -> w312 mode=indexing
            i -> [w315]
          }
          n165 = Build Array(w311, w309) -> (w310:string[][])
          n166 = Transpose 2D Array(2D array=w310) -> (transposed array=w313:string[][])
          n167 = Number To Decimal String(number=w312) -> (decimal integer string=w314:string[])  [unwired: 1 in]
        }
      }
      n168 = property on="多列列表框" class="MCListbox (严格)"("ItemNames"=w298, "RowHdrs[]"=w299) -> ()  [unwired: 2 in, 2 out]
    }
  }
  n169 = Obtain Notifier(name (unnamed)="NH3N" ("名称（未命名）"), notification data type=FALSE) -> (notifier out=w3:refnum<notifier>)  [unwired: 2 in, 2 out]
  n170 = Obtain Queue(name (unnamed)="NH3N" ("名称（未命名）"), element data type=cluster{"命令":string, "data":variant} {"命令"="", "data"=variant}) -> (queue out=w17:refnum<queue>, error out=w18:errorcluster)  [unwired: 3 in, 1 out]
  n171 = while {
    tunnel: w6 -> [w331]
    tunnel: [w328] -> _
    stop <- FALSE stop-if-true
    w332 = u16 3 items=["总磷"=1, "氨氮"=3] ("站号")
    # "定时更新"
    n172 = Wait (ms)(milliseconds to wait=u32 30000 ("等待时间（毫秒）")) -> ()  [unwired: 1 out]
    n173 = call "氨氮版本号读取.vi"() -> ("error out"=w328:errorcluster, "固件版本号"=→"固件版本号":string)  [unwired: 10 in]
    n174 = Bundle By Name(cluster=cluster{"命令":string, "data":variant} {"命令"="", "data"=variant} ("元素"), "命令"="读序列号", "data"=w332) -> (w330:cluster{"命令":string, "data":variant})
    n175 = Enqueue Element(queue=w331, element=w330) -> ()  [unwired: 2 in, 3 out]
  }
  n176 = control-ref of="测量模式下拉列表"() -> (w13:refnum<vi>)
  n177 = control-ref of="量程切换阈值"() -> (w11:refnum<vi>)
  n178 = control-ref of="参数下拉列表"() -> (w14:refnum<vi>)
  n179 = control-ref of="量程下拉列表"() -> (w15:refnum<vi>)
  n180 = control-ref of="备用系数"() -> (w10:refnum<vi>)
  n181 = control-ref of="公式"() -> (w12:refnum<vi>)
  n182 = while {
    tunnel: w17 -> [w354]
    tunnel: w18 -> [_]
    shift-right: [w348] -> _
    shift-left: enum16{"氨氮", "总磷"}."氨氮" ("枚举") -> [w349]
    stop <- FALSE stop-if-true
    w347 = u16 3 items=["总磷"=1, "氨氮"=3] ("站号")
    # "试剂填充 172 \n管路清洗108\n氨氮92\n总磷131\n总磷海水147\n总氮76\n总氮海水92"
    n183 = Wait (ms)(milliseconds to wait=u32 1000 ("等待时间（毫秒）")) -> ()  [unwired: 1 out]
    n184 = global read "氨氮断电保存全局变量.vi" "流程文件路径"() -> (w336:path)
    n185 = global read "VAR氨氮全局变量.vi" "状态告警区"() -> (w345:T4)
    n186 = Bundle By Name(cluster=cluster{"命令":string, "data":variant} {"命令"="", "data"=variant} ("元素"), "命令"="读状态告警区", "data"=w347) -> (w356:cluster{"命令":string, "data":variant})
    n187 = local write "流程文件路径"(w336) -> ()
    n188 = Bundle By Name(cluster=cluster{"命令":string, "data":variant} {"命令"="", "data"=variant} ("元素"), "命令"="读测量数据区", "data"=w347) -> (w352:cluster{"命令":string, "data":variant})
    n189 = Unbundle By Name(w345) -> ("系统时间"=w344:timestamp)
    n190 = Enqueue Element(queue=w354, element=w356) -> (queue out=w350:refnum<queue>)  [unwired: 2 in, 2 out]
    n191 = Enqueue Element(queue=w350, element=w352) -> (queue out=w346:refnum<queue>)  [unwired: 2 in, 2 out]
    n192 = Get Date/Time In Seconds() -> (seconds since 1Jan1904=w343:timestamp)
    n193 = Subtract(x=w343, y=w344) -> (x-y=w342:dbl)
    n194 = Absolute Value(x=w342) -> (abs(x)=w341:dbl)
    n195 = global read "VAR氨氮全局变量.vi" "通讯状态"() -> (w337:bool)
    n196 = Greater Or Equal?(x=w341, y=120.0) -> (x >= y?=w339:bool)
    n197 = And(x=w337, y=w339) -> (x .and. y?=w338:bool)
    n198 = case shown="真" w338 {
      tunnel: w346 -> [_ w361]
      frame False {
      }
      frame True {
        n199 = call "氨氮启动命令.vi"("参数"=T5 {"站号"=3, "量程切换"=enum."AUTO", "控制命令"=enum."校时", "模式设置"=enum."待机", "测量间隔"=0}) -> ("启动命令"=w360:cluster{"命令":string, "data":variant})  [unwired: 10 in]
        n200 = Enqueue Element(queue=w361, element=w360) -> ()  [unwired: 2 in, 3 out]
      }
    }
    n201 = Increment(x=w349) -> (x+1=w348:enum16{"氨氮", "总磷"})
  }
  n202 = while {
    tunnel: w17 -> [w370]
    tunnel: w15 -> [w369]
    tunnel: w14 -> [w368]
    tunnel: w13 -> [w367]
    tunnel: w12 -> [w366]
    tunnel: w11 -> [w365]
    tunnel: w10 -> [w364]
    tunnel: w3 -> [w363]
    tunnel: w2 -> [_]
    stop <- FALSE stop-if-true
    n203 = event shown="[2] \"模块启用\": 值改变" {
      selector: _ -> [_ _ _ _ _ _ _ _ _ _ _ _ _ _ _ _ _ _ _ _ _ _]
      dyn-events: _ -> [_ _ _ _ _ _ _ _ _ _ _ _ _ _ _ _ _ _ _ _ _ _]
      timeout: _ -> [_ _ _ _ _ _ _ _ _ _ _ _ _ _ _ _ _ _ _ _ _ _]
      tunnel: w370 -> [_ w372 w395 _ _ _ _ _ _ w462 _ w487 w492 _ _ _ _ _ _ _ _ _]
      tunnel: w369 -> [_ _ _ _ _ _ _ _ _ _ _ _ _ _ _ _ w508 _ w528 w537 w544 w555]
      tunnel: w368 -> [_ _ _ _ _ _ _ _ _ _ _ _ _ _ _ _ w506 _ w526 w539 w551 w562]
      tunnel: w367 -> [_ _ _ _ _ _ _ _ _ _ _ _ _ _ _ _ w507 _ w527 w538 w545 w557]
      tunnel: w366 -> [_ _ _ _ _ _ _ _ _ _ _ _ _ _ _ _ w502 _ _ _ _ _]
      tunnel: w365 -> [_ _ _ _ _ _ _ _ _ _ _ _ _ _ _ _ _ _ w522 _ _ _]
      tunnel: w364 -> [_ _ _ _ _ _ _ _ _ _ _ _ _ _ _ _ _ _ _ _ w549 _]
      tunnel: w363 -> [_ _ _ _ _ _ _ _ _ _ _ _ w490 _ _ _ _ _ _ _ _ _]
      event Timeout {
        n204 = event-data() -> ()  [unwired: 1 in, 3 out]
      }
      event "串口设置": Value Change {
        n205 = event-data() -> ()  [unwired: 1 in, 6 out]
        n206 = global read "氨氮断电保存全局变量.vi" "VISA Resource"() -> (w375:refnum<visa-resource-name>)
        n207 = call "串口配置.vi"("VISA资源名称"=w375) -> ("确认 2"=w374:bool, "VISA资源名称 2"=w373:refnum<visa-resource-name>)  [unwired: 9 in]
        n208 = case shown="真" w374 {
          tunnel: w373 -> [_ w377]
          tunnel: w372 -> [_ w376]
          frame False {
          }
          frame True {
            n209 = flat-sequence {
              tunnel: w377 -> [w380]
              tunnel: w376 -> [w378]
              frame #0 {
                n210 = global write "氨氮断电保存全局变量.vi" "VISA Resource"(w380) -> ()
                n211 = Enqueue Element(queue=w378, element=cluster{"命令":string, "data":variant} {"命令"="启用模块", "data"=variant} ("元素")) -> ()  [unwired: 2 in, 3 out]
              }
              frame #1 {
                n212 = call <vilib>:"Application Directory.vi"() -> ("Application Directory"=w394:path)
                n213 = Build Path(base path=w394, name or relative path="data\\sys.ini" ("名称或相对路径")) -> (appended path=w392:path)
                n214 = call <vilib>:"Open Config Data.vi"("configuration file path"=w392) -> ("error out"=w388:errorcluster, "refnum"=w391:T13)  [unwired: 8 in, 1 out]
                n215 = vi-ref "氨氮断电保存全局变量.vi"() -> (w390:refnum<vi>)
                n216 = call <userlib>:"Write Panel to INI__ogtk.vi"("error in (no error)"=w388, "VI ref"=w390, "refnum"=w391) -> ("error out"=w387:errorcluster, "refnum out"=w389:T13)  [unwired: 7 in]
                n217 = call <vilib>:"Close Config Data.vi"("error in (no error)"=w387, "refnum"=w389) -> ("error out"=w382:errorcluster, "file path"=w381:path)  [unwired: 8 in]
                n218 = Open/Create/Replace File(file path (use dialog)=w381, error in=w382) -> (refnum out=w385:refnum<file>, error out=w386:errorcluster)  [unwired: 4 in, 1 out]
                n219 = Flush File(refnum=w385, error in=w386) -> (refnum out=w384:refnum<file>, error out=w383:errorcluster)
                n220 = Close File(refnum=w384, error in=w383) -> ()  [unwired: 2 out]
              }
            }
          }
        }
      }
      event "模块启用": Value Change {
        n221 = event-data() -> ("OldVal"=w396:bool)  [unwired: 1 in, 5 out]
        n222 = case shown="假" w396 {
          tunnel: w395 -> [w397 w399]
          frame False {
            n223 = Enqueue Element(queue=w397, element=cluster{"命令":string, "data":variant} {"命令"="停用模块", "data"=variant} ("元素")) -> ()  [unwired: 2 in, 3 out]
          }
          frame True {
            n224 = Enqueue Element(queue=w399, element=cluster{"命令":string, "data":variant} {"命令"="启用模块", "data"=variant} ("元素")) -> ()  [unwired: 2 in, 3 out]
          }
        }
      }
      event "流程文件路径": Value Change {
        n225 = event-data() -> ()  [unwired: 1 in, 6 out]
        n226 = flat-sequence {
          frame #0 {
            n227 = local read "流程文件路径"() -> (w401:path)
            n228 = global write "氨氮断电保存全局变量.vi" "流程文件路径"(w401) -> ()
          }
          frame #1 {
            n229 = call <vilib>:"Application Directory.vi"() -> ("Application Directory"=w415:path)
            n230 = Build Path(base path=w415, name or relative path="data\\sys.ini" ("名称或相对路径")) -> (appended path=w413:path)
            n231 = call <vilib>:"Open Config Data.vi"("configuration file path"=w413) -> ("error out"=w409:errorcluster, "refnum"=w412:T13)  [unwired: 8 in, 1 out]
            n232 = vi-ref "氨氮断电保存全局变量.vi"() -> (w411:refnum<vi>)
            n233 = call <userlib>:"Write Panel to INI__ogtk.vi"("error in (no error)"=w409, "VI ref"=w411, "refnum"=w412) -> ("error out"=w408:errorcluster, "refnum out"=w410:T13)  [unwired: 7 in]
            n234 = call <vilib>:"Close Config Data.vi"("error in (no error)"=w408, "refnum"=w410) -> ("error out"=w403:errorcluster, "file path"=w402:path)  [unwired: 8 in]
            n235 = Open/Create/Replace File(file path (use dialog)=w402, error in=w403) -> (refnum out=w406:refnum<file>, error out=w407:errorcluster)  [unwired: 4 in, 1 out]
            n236 = Flush File(refnum=w406, error in=w407) -> (refnum out=w405:refnum<file>, error out=w404:errorcluster)
            n237 = Close File(refnum=w405, error in=w404) -> ()  [unwired: 2 out]
          }
        }
      }
      event "公式一键写入": Value Change {
        n238 = event-data() -> ()  [unwired: 1 in, 6 out]
        n239 = local read "公式"() -> (w416:cluster{"X^2":dbl, "X":dbl, "b":dbl})
        n240 = call "公式复合写入.vi"("公式"=w416) -> ()  [unwired: 11 in]
      }
      event "备用系数一键写入": Value Change {
        n241 = event-data() -> ()  [unwired: 1 in, 6 out]
        n242 = local read "备用系数"() -> (w417:T2)
        n243 = call "量程参数复合参数写入.vi"("备用系数"=w417) -> ()  [unwired: 11 in]
      }
      event "曲线模型": Value Change {
        n244 = event-data() -> ()  [unwired: 1 in, 6 out]
        n245 = local write "公式"("曲线模型") -> ()
      }
      event "质控参数设置": Value Change {
        n246 = event-data() -> ()  [unwired: 1 in, 6 out]
        n247 = global read "氨氮断电保存全局变量.vi" "质控参数设置"() -> (w419:T19)
        n248 = call "质控参数设置.vi"("质控参数设置"=w419) -> ("输出簇"=w420:T20)  [unwired: 10 in]
        n249 = Unbundle By Name(w420) -> ("确定"=w421:bool)
        n250 = case shown="真" w421 {
          tunnel: w420 -> [_ w423]
          tunnel: w419 -> [_ w422]
          frame False {
          }
          frame True {
            n251 = flat-sequence {
              tunnel: w423 -> [w430]
              tunnel: w422 -> [w424]
              frame #0 {
                n252 = Unbundle By Name(w430) -> ("跨度值"=w429:dbl, "零点标准液浓度"=w428:dbl, "跨度标准液浓度"=w427:dbl, "标准液标准浓度"=w426:dbl)
                n253 = Bundle By Name(cluster=w424, "跨度值"=w429, "零点标准液浓度"=w428, "跨度标准液浓度"=w427, "标准液标准浓度"=w426) -> (w425:T19)
                n254 = global write "氨氮断电保存全局变量.vi" "质控参数设置"(w425) -> ()
              }
              frame #1 {
                n255 = call <vilib>:"Application Directory.vi"() -> ("Application Directory"=w431:path)
                n256 = Build Path(base path=w431, name or relative path="data\\sys.ini" ("名称或相对路径")) -> (appended path=w433:path)
                n257 = call <vilib>:"Open Config Data.vi"("configuration file path"=w433) -> ("error out"=w437:errorcluster, "refnum"=w434:T13)  [unwired: 8 in, 1 out]
                n258 = vi-ref "氨氮断电保存全局变量.vi"() -> (w435:refnum<vi>)
                n259 = call <userlib>:"Write Panel to INI__ogtk.vi"("error in (no error)"=w437, "VI ref"=w435, "refnum"=w434) -> ("error out"=w438:errorcluster, "refnum out"=w436:T13)  [unwired: 7 in]
                n260 = call <vilib>:"Close Config Data.vi"("error in (no error)"=w438, "refnum"=w436) -> ("error out"=w443:errorcluster, "file path"=w444:path)  [unwired: 8 in]
                n261 = Open/Create/Replace File(file path (use dialog)=w444, error in=w443) -> (refnum out=w440:refnum<file>, error out=w439:errorcluster)  [unwired: 4 in, 1 out]
                n262 = Flush File(refnum=w440, error in=w439) -> (refnum out=w441:refnum<file>, error out=w442:errorcluster)
                n263 = Close File(refnum=w441, error in=w442) -> ()  [unwired: 2 out]
              }
            }
          }
        }
      }
      event "氨氮自动测试量程配置": Value Change {
        n264 = event-data() -> ()  [unwired: 1 in, 6 out]
        n265 = flat-sequence {
          frame #0 {
            n266 = global write "氨氮断电保存全局变量.vi" "氨氮自动测试量程配置"("氨氮自动测试量程配置") -> ()
          }
          frame #1 {
            n267 = call <vilib>:"Application Directory.vi"() -> ("Application Directory"=w459:path)
            n268 = Build Path(base path=w459, name or relative path="data\\sys.ini" ("名称或相对路径")) -> (appended path=w457:path)
            n269 = call <vilib>:"Open Config Data.vi"("configuration file path"=w457) -> ("error out"=w453:errorcluster, "refnum"=w456:T13)  [unwired: 8 in, 1 out]
            n270 = vi-ref "氨氮断电保存全局变量.vi"() -> (w455:refnum<vi>)
            n271 = call <userlib>:"Write Panel to INI__ogtk.vi"("error in (no error)"=w453, "VI ref"=w455, "refnum"=w456) -> ("error out"=w452:errorcluster, "refnum out"=w454:T13)  [unwired: 7 in]
            n272 = call <vilib>:"Close Config Data.vi"("error in (no error)"=w452, "refnum"=w454) -> ("error out"=w447:errorcluster, "file path"=w446:path)  [unwired: 8 in]
            n273 = Open/Create/Replace File(file path (use dialog)=w446, error in=w447) -> (refnum out=w450:refnum<file>, error out=w451:errorcluster)  [unwired: 4 in, 1 out]
            n274 = Flush File(refnum=w450, error in=w451) -> (refnum out=w449:refnum<file>, error out=w448:errorcluster)
            n275 = Close File(refnum=w449, error in=w448) -> ()  [unwired: 2 out]
          }
        }
      }
      event "手动启动": Value Change {
        n276 = event-data() -> ()  [unwired: 1 in, 6 out]
        n277 = call "氨氮启动参数对话框.vi"() -> ("确认"=w460:bool, "元素"=w461:cluster{"命令":string, "data":variant})  [unwired: 10 in]
        n278 = case shown="真" w460 {
          tunnel: w462 -> [_ w464]
          tunnel: w461 -> [_ w463]
          frame False {
          }
          frame True {
            n279 = Enqueue Element(queue=w464, element=w463) -> ()  [unwired: 2 in, 3 out]
          }
        }
      }
      event "定时启动": Mouse Down {
        n280 = event-data() -> ()  [unwired: 1 in, 6 out]
        n281 = flat-sequence {
          frame #0 {
            n282 = global read "氨氮断电保存全局变量.vi" "定时控制"() -> (w465:T7)
            n283 = call "周期设置.vi"("定时控制参数输入"=w465) -> ("定时控制参数输出"=w466:T7)  [unwired: 10 in]
            n284 = global write "氨氮断电保存全局变量.vi" "定时控制"(w466) -> ()
          }
          frame #1 {
            n285 = call <vilib>:"Application Directory.vi"() -> ("Application Directory"=w480:path)
            n286 = Build Path(base path=w480, name or relative path="data\\sys.ini" ("名称或相对路径")) -> (appended path=w478:path)
            n287 = call <vilib>:"Open Config Data.vi"("configuration file path"=w478) -> ("error out"=w474:errorcluster, "refnum"=w477:T13)  [unwired: 8 in, 1 out]
            n288 = vi-ref "氨氮断电保存全局变量.vi"() -> (w476:refnum<vi>)
            n289 = call <userlib>:"Write Panel to INI__ogtk.vi"("error in (no error)"=w474, "VI ref"=w476, "refnum"=w477) -> ("error out"=w473:errorcluster, "refnum out"=w475:T13)  [unwired: 7 in]
            n290 = call <vilib>:"Close Config Data.vi"("error in (no error)"=w473, "refnum"=w475) -> ("error out"=w468:errorcluster, "file path"=w467:path)  [unwired: 8 in]
            n291 = Open/Create/Replace File(file path (use dialog)=w467, error in=w468) -> (refnum out=w471:refnum<file>, error out=w472:errorcluster)  [unwired: 4 in, 1 out]
            n292 = Flush File(refnum=w471, error in=w472) -> (refnum out=w470:refnum<file>, error out=w469:errorcluster)
            n293 = Close File(refnum=w470, error in=w469) -> ()  [unwired: 2 out]
          }
        }
      }
      event "单步测试": Value Change {
        w482 = u16 1 items=["总磷"=1, "氨氮"=3] ("站号")
        n294 = event-data() -> ()  [unwired: 1 in, 6 out]
        n295 = Bundle("站号"=w482, "总磷氨氮调试"="总磷氨氮调试") -> (w481:cluster{"站号":u16, "总磷氨氮调试":u16[]})  [unwired: 1 in]
        n296 = Bundle By Name(cluster=cluster{"命令":string, "data":variant} {"命令"="", "data"=variant} ("元素"), "命令"="debug", "data"=w481) -> (w484:cluster{"命令":string, "data":variant})
        n297 = Enqueue Element(queue=w487, element=w484) -> ()  [unwired: 2 in, 3 out]
      }
      event "停止": Value Change {
        n298 = event-data() -> ()  [unwired: 1 in, 6 out]
        n299 = Enqueue Element(queue=w492, element=cluster{"命令":string, "data":variant} {"命令"="启动", "data"=variant(cluster{"站号":u16, "控制命令输出":u16[]} {"站号"=3, "控制命令输出"=[2816]})} ("启动命令")) -> ()  [unwired: 2 in, 3 out]
        n300 = Cancel Notification(0:w490) -> (8:w489:refnum<notifier>)  [unwired: 1 in, 2 out]
        n301 = Send Notification(notification=TRUE ("通知"), notifier=w489) -> ()  [unwired: 1 in, 2 out]
      }
      event "设置": Value Change {
        n302 = event-data() -> ()  [unwired: 1 in, 6 out]
        n303 = property on="窗格" class="Pane"("Origin"=T10 {"Horizontal"=0, "Vertical"=628} ("原点")) -> ()  [unwired: 2 in, 2 out]
      }
      event "返回": Value Change {
        n304 = event-data() -> ()  [unwired: 1 in, 6 out]
        n305 = property on="窗格" class="Pane"("Origin"=T10 {"Horizontal"=0, "Vertical"=0} ("原点")) -> ()  [unwired: 2 in, 2 out]
      }
      event "公式.X^2", "公式.X", "公式.b", "量程切换阈值.阈值", "量程切换阈值.标液浓度", "备用系数.量程上限", "备用系数.量程下限", "备用系数.检出限", "备用系数.精度": Mouse Down {
        n306 = event-data() -> ("CtlRef"=w498:refnum<vi>)  [unwired: 1 in, 5 out]
        n307 = property class="DigNum (严格)"(reference=w498) -> (reference out=w496:refnum<vi>, "Value"=w497:dbl)  [unwired: 1 in, 1 out]
        n308 = call "数字键盘.vi"("OldNumber"=w497) -> ("NewNumber"=w495:dbl)
        n309 = property class="DigNum (严格)"(reference=w496, "Val(Sgnl)"=w495) -> ()  [unwired: 1 in, 2 out]
      }
      event "读公式": Value Change {
        n310 = event-data() -> ()  [unwired: 1 in, 6 out]
        n311 = property class="Enum (严格)"(reference=w506) -> ("Value"=w505:enum16{"氨氮", "总磷"})  [unwired: 1 in, 2 out]
        n312 = property class="Enum (严格)"(reference=w507) -> ("Value"=w504:enum16{"水样测量", "空白核查", "跨度核查", "标样核查", "加标回收"})  [unwired: 1 in, 2 out]
        n313 = property class="Enum (严格)"(reference=w508) -> ("Value"=w503:enum16{"低量程", "高量程"})  [unwired: 1 in, 2 out]
        n314 = call "氨氮公式读取.vi"("量程"=w503, "测量模式"=w504, "测量参数"=w505) -> ("error out"=w500:errorcluster, "公式"=w501:cluster{"X^2":dbl, "X":dbl, "b":dbl})  [unwired: 7 in]
        n315 = property class="Clust (严格)"(reference=w502, "Value"=w501) -> ()  [unwired: 1 in, 2 out]
        n316 = case shown="错误" w500 {
          tunnel: ["读取成功" ("消息") "读取失败" ("消息")] -> w499
          frame No Error {
          }
          frame Error {
          }
        }
        n317 = One Button Dialog(message=w499) -> ()  [unwired: 1 in, 1 out]
      }
      event "写公式": Value Change {
        n318 = event-data() -> ()  [unwired: 1 in, 6 out]
        n319 = call "氨氮公式写入.vi"("公式"="公式", "量程"="量程下拉列表", "测量模式"="测量模式下拉列表", "测量参数"="参数下拉列表") -> ("error out"=w511:errorcluster)  [unwired: 7 in]
        n320 = case shown="无错误" w511 {
          tunnel: ["写入成功" ("消息") "写入失败" ("消息")] -> w512
          frame No Error {
          }
          frame Error {
          }
        }
        n321 = One Button Dialog(message=w512) -> ()  [unwired: 1 in, 1 out]
      }
      event "量程切换阈值读取": Value Change {
        n322 = event-data() -> ()  [unwired: 1 in, 6 out]
        n323 = property class="Enum (严格)"(reference=w526) -> ("Value"=w525:enum16{"氨氮", "总磷"})  [unwired: 1 in, 2 out]
        n324 = property class="Enum (严格)"(reference=w527) -> ("Value"=w524:enum16{"水样测量", "空白核查", "跨度核查", "标样核查", "加标回收"})  [unwired: 1 in, 2 out]
        n325 = property class="Enum (严格)"(reference=w528) -> ("Value"=w523:enum16{"低量程", "高量程"})  [unwired: 1 in, 2 out]
        n326 = call "氨氮量程读取.vi"("量程"=w523, "测量模式"=w524, "测量参数"=w525) -> ("error out"=w519:errorcluster, "量程切换阈值"=w521:cluster{"阈值":dbl, "标液浓度":dbl})  [unwired: 7 in]
        n327 = property class="Clust (严格)"(reference=w522, "Value"=w521) -> ()  [unwired: 1 in, 2 out]
        n328 = case shown="错误" w519 {
          tunnel: ["读取成功" ("消息") "读取失败" ("消息")] -> w520
          frame No Error {
          }
          frame Error {
          }
        }
        n329 = One Button Dialog(message=w520) -> ()  [unwired: 1 in, 1 out]
      }
      event "量程切换阈值写入": Value Change {
        n330 = event-data() -> ()  [unwired: 1 in, 6 out]
        n331 = property class="Enum (严格)"(reference=w539) -> ("Value"=w536:enum16{"氨氮", "总磷"})  [unwired: 1 in, 2 out]
        n332 = property class="Enum (严格)"(reference=w538) -> ("Value"=w535:enum16{"水样测量", "空白核查", "跨度核查", "标样核查", "加标回收"})  [unwired: 1 in, 2 out]
        n333 = property class="Enum (严格)"(reference=w537) -> ("Value"=w534:enum16{"低量程", "高量程"})  [unwired: 1 in, 2 out]
        n334 = call "氨氮量程写入.vi"("量程切换阈值"="量程切换阈值", "量程"=w534, "测量模式"=w535, "测量参数"=w536) -> ("error out"=w531:errorcluster)  [unwired: 7 in]
        n335 = case shown="无错误" w531 {
          tunnel: ["写入成功" ("消息") "写入失败" ("消息")] -> w532
          frame No Error {
          }
          frame Error {
          }
        }
        n336 = One Button Dialog(message=w532) -> ()  [unwired: 1 in, 1 out]
      }
      event "备用系数读取": Value Change {
        n337 = event-data() -> ()  [unwired: 1 in, 6 out]
        n338 = property class="Enum (严格)"(reference=w551) -> ("Value"=w550:enum16{"氨氮", "总磷"})  [unwired: 1 in, 2 out]
        n339 = property class="Enum (严格)"(reference=w545) -> ("Value"=w542:enum16{"水样测量", "空白核查", "跨度核查", "标样核查", "加标回收"})  [unwired: 1 in, 2 out]
        n340 = property class="Enum (严格)"(reference=w544) -> ("Value"=w543:enum16{"低量程", "高量程"})  [unwired: 1 in, 2 out]
        n341 = call "氨氮备用系数读取.vi"("量程"=w543, "测量模式"=w542, "测量参数"=w550) -> ("error out"=w546:errorcluster, "备用系数"=w548:T2)  [unwired: 7 in]
        n342 = property class="Clust (严格)"(reference=w549, "Value"=w548) -> ()  [unwired: 1 in, 2 out]
        n343 = case shown="错误" w546 {
          tunnel: ["读取成功" ("消息") "读取失败" ("消息")] -> w547
          frame No Error {
          }
          frame Error {
          }
        }
        n344 = One Button Dialog(message=w547) -> ()  [unwired: 1 in, 1 out]
      }
      event "备用系数写入": Value Change {
        n345 = event-data() -> ()  [unwired: 1 in, 6 out]
        n346 = property class="Enum (严格)"(reference=w562) -> ("Value"=w561:enum16{"氨氮", "总磷"})  [unwired: 1 in, 2 out]
        n347 = property class="Enum (严格)"(reference=w557) -> ("Value"=w556:enum16{"水样测量", "空白核查", "跨度核查", "标样核查", "加标回收"})  [unwired: 1 in, 2 out]
        n348 = property class="Enum (严格)"(reference=w555) -> ("Value"=w554:enum16{"低量程", "高量程"})  [unwired: 1 in, 2 out]
        n349 = call "氨氮备用系数写入.vi"("备用系数"="备用系数", "量程"=w554, "测量模式"=w556, "测量参数"=w561) -> ("error out"=w558:errorcluster)  [unwired: 7 in]
        n350 = case shown="无错误" w558 {
          tunnel: ["写入成功" ("消息") "写入失败" ("消息")] -> w559
          frame No Error {
          }
          frame Error {
          }
        }
        n351 = One Button Dialog(message=w559) -> ()  [unwired: 1 in, 1 out]
      }
    }
  }
